vi "IsGoalReached.vi"(8 "error in":errorcluster, 9 "RobotPosition":cluster{"X":dbl, "Y":dbl, "Angle":dbl}, 10 "Goal":T1) -> (0 "error out":errorcluster, 2 "Reached":bool)   [LabVIEW 2009, in "Main.lvlib"]
uses:
  Main.lvlib
  Drive/Drive_Point.ctl
  Drive/Drive_Utils.lvlib
  Drive.lvlib
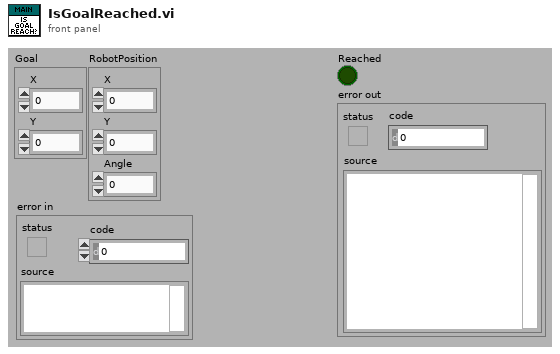
[diagram p1: front panel]
types:
  T1 = typedef "Drive.lvlib/Drive_Point.ctl" = cluster{"X":dbl, "Y":dbl}
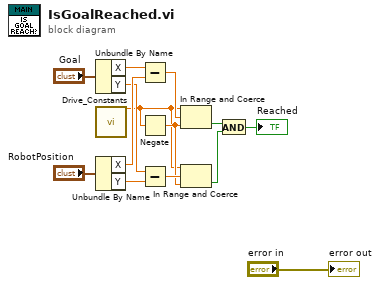
[diagram p0: block diagram]
diagram:
  n1 = Unbundle By Name("Goal") -> ("X"=w11:dbl, "Y"=w9:dbl)
  n2 = call "Drive_Constants.vi"() -> ("Position accuracy (m)"=w5:dbl)  [unwired: 19 in, 8 out]
  n3 = Unbundle By Name("RobotPosition") -> ("X"=w10:dbl, "Y"=w8:dbl)
  n4 = Subtract(x=w11, y=w10) -> (x-y=w12:dbl)
  n5 = Negate(x=w5) -> (-x=w6:dbl)
  n6 = Subtract(x=w9, y=w8) -> (x-y=w7:dbl)
  n7 = In Range and Coerce(upper limit=w5, x=w12, lower limit=w6) -> (In Range?=w14:bool)  [unwired: 1 out]
  n8 = In Range and Coerce(upper limit=w5, x=w7, lower limit=w6) -> (In Range?=w13:bool)  [unwired: 1 out]
  n9 = And(x=w14, y=w13) -> (x .and. y?=→"Reached":bool)
  "error out" <- "error in"
